vi "SCT Start Attributes Message.vi"(4 "main loop broadcast listener":T7, 6 "feature pack info":T8, 8 "error in (no error)":errorcluster, 9 "Event Registration Refnum":refnum<event-registration>, 10 "state variables in":T2, 11 "Variable Dialog Controls":T1) -> (0 "error out":errorcluster, 1 "Event Registration Refnum 2":refnum<event-registration>, 2 "state variables out":T2, 3 "Variable Dialog Controls out":T1, 5 "done?":bool)   [LabVIEW 2016]
uses:
  <resource>/dialog/variable/SCT Variable Dialog Controls.ctl
  <resource>/dialog/variable/SCT Feature Pack Info.ctl
  <resource>/dialog/variable/SCT Message User Event.ctl
  <resource>/dialog/variable/SCT Message.ctl
  <vilib>/variable/Type Descriptor.ctl
  <resource>/dialog/variable/SCT Attributes.ctl
  <resource>/dialog/variable/SCT Attributes Event.ctl
  <resource>/dialog/variable/SCT Broadcast User Event.ctl
  <resource>/dialog/variable/SCT Broadcast.ctl
  <resource>/dialog/variable/SCT State Variables.ctl
  <resource>/dialog/variable/SCT Feature State.ctl
  <resource>/dialog/variable/SCT Variable Changes.ctl
  <resource>/dialog/variable/SCT Attribute Changes.ctl
  <vilib>/variable/NI_Variable.lvlib
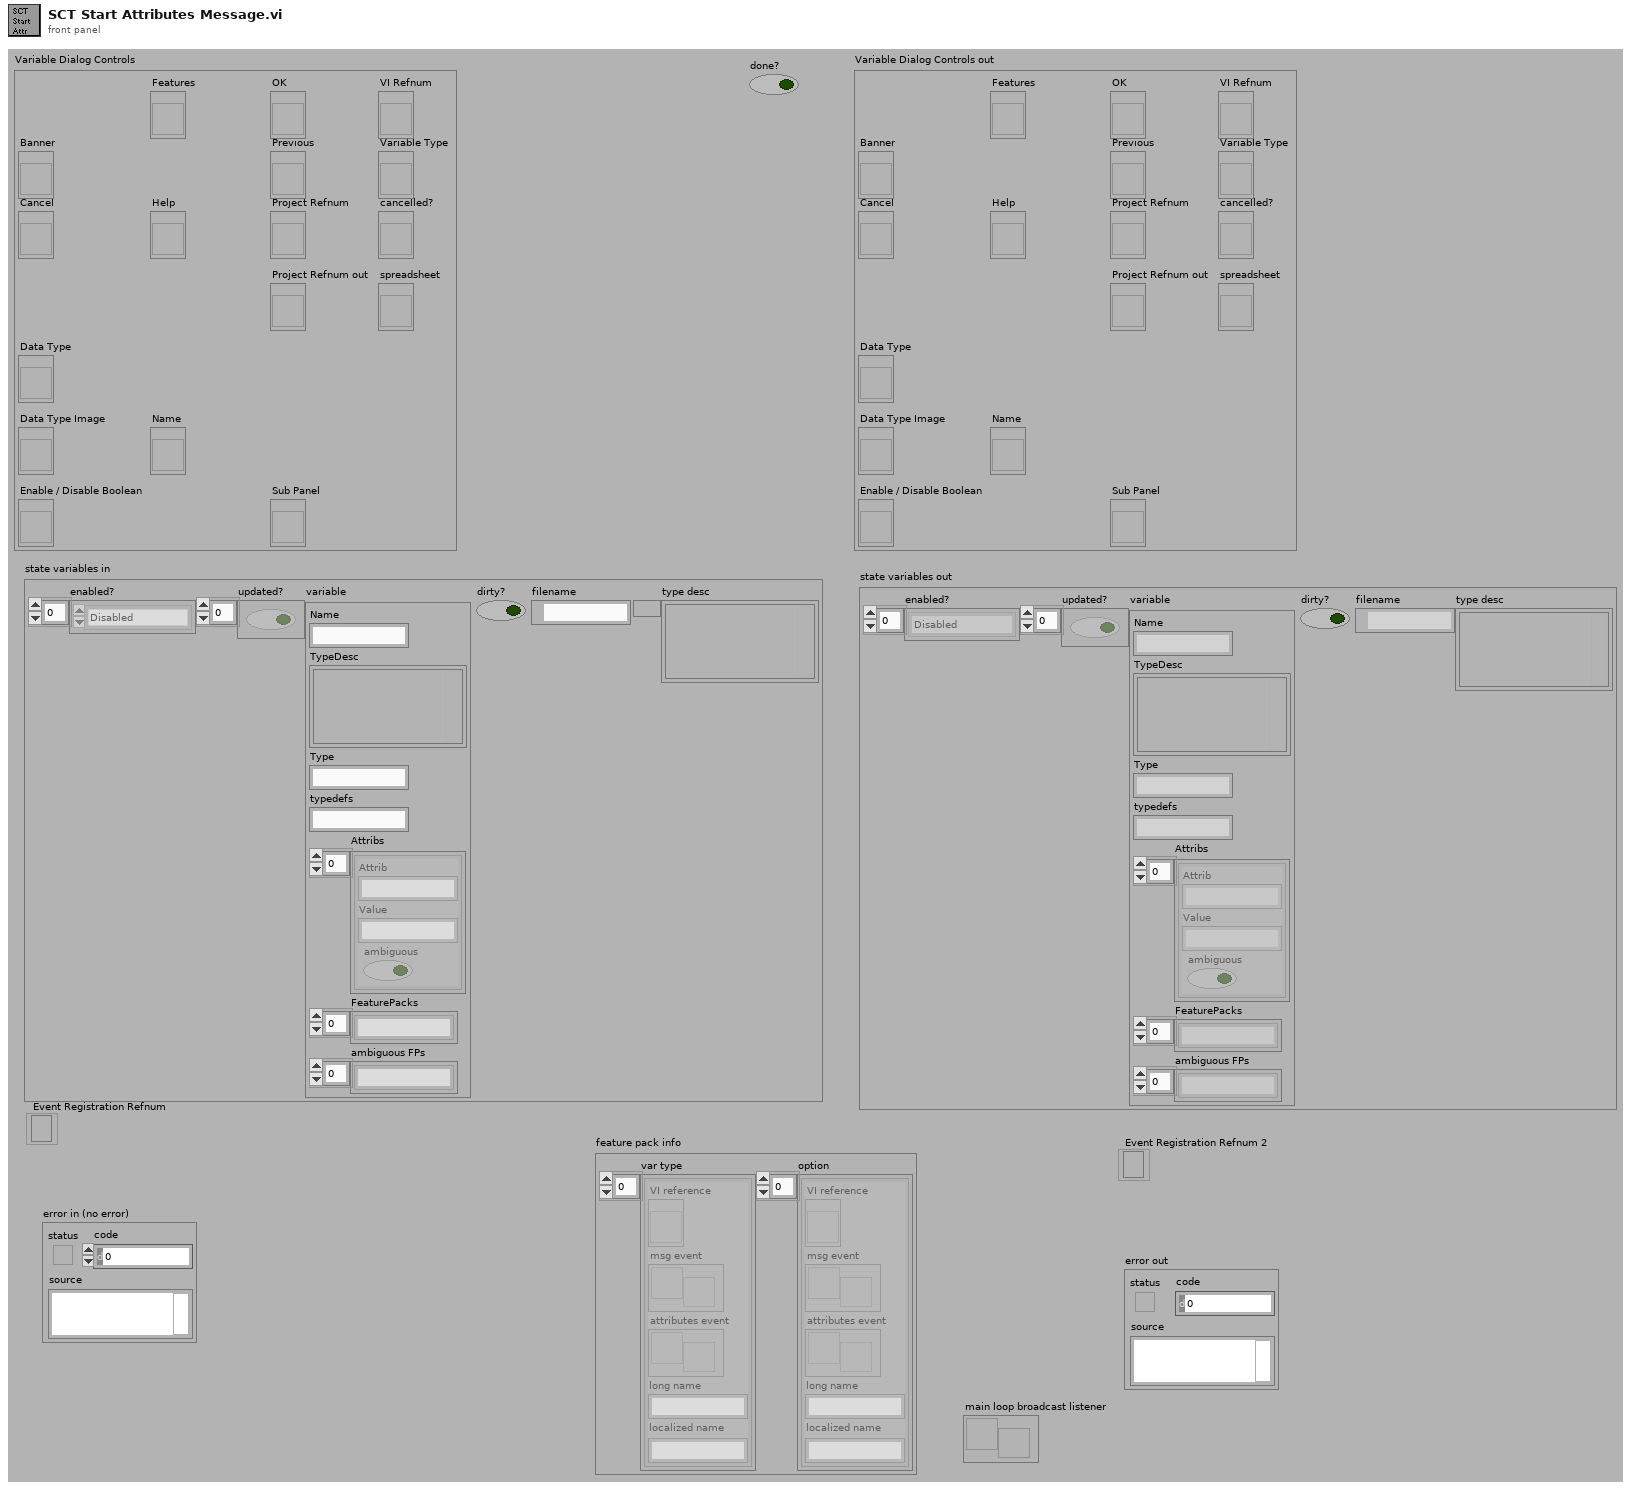
[diagram p1: front panel]
types:
  T1 = typedef "SCT Variable Dialog Controls.ctl" = cluster{"Banner":refnum<vi>, "Cancel":refnum<vi>, "Data Type":refnum<vi>, "Data Type Image":refnum<vi>, "Enable / Disable Boolean":refnum<vi>, "Features":refnum<vi>, "Help":refnum<vi>, "Name":refnum<vi>, "OK":refnum<vi>, "Previous":refnum<vi>, "Project Refnum":refnum<vi>, "Project Refnum out":refnum<vi>, "Sub Panel":refnum<vi>, "VI Refnum":refnum<vi>, "Variable Type":refnum<vi>, "cancelled?":refnum<vi>, "spreadsheet":refnum<vi>}
  T2 = typedef "SCT State Variables.ctl" = cluster{"enabled?":T3[], "updated?":bool[], "variable":T4, "dirty?":bool, "filename":path, "type desc":T5}
  T3 = typedef "SCT Feature State.ctl" = enum16{"Disabled", "Enabled", "Ambiguous", "Grayed", "MultiSelectConst"}
  T4 = typedef "SCT Variable Changes.ctl" = cluster{"Name":string, "TypeDesc":T5, "Type":string, "typedefs":string, "Attribs":T6, "FeaturePacks":string[], "ambiguous FPs":string[]}
  T5 = typedef "NI_Variable.lvlib/Type Descriptor.ctl" = cluster{"Variant":variant}
  T6 = typedef "SCT Attribute Changes.ctl" = cluster{"Attrib":string, "Value":string, "ambiguous":bool}[]
  T7 = typedef "SCT Broadcast User Event.ctl" = refnum<user-event>
  T8 = typedef "SCT Feature Pack Info.ctl" = cluster{"var type":cluster{"VI reference":refnum<vi>, "msg event":T9, "attributes event":T10, "long name":string, "localized name":string}[], "option":cluster{"VI reference":refnum<vi>, "msg event":T9, "attributes event":T10, "long name":string, "localized name":string}[]}
  T9 = typedef "SCT Message User Event.ctl" = refnum<user-event>
  T10 = typedef "SCT Attributes Event.ctl" = refnum<user-event>
  T11 = cluster{"VI reference":refnum<vi>, "msg event":T9, "attributes event":T10, "long name":string, "localized name":string}[]
  T12 = cluster{"VI reference":refnum<vi>, "msg event":T9, "attributes event":T10, "long name":string, "localized name":string}
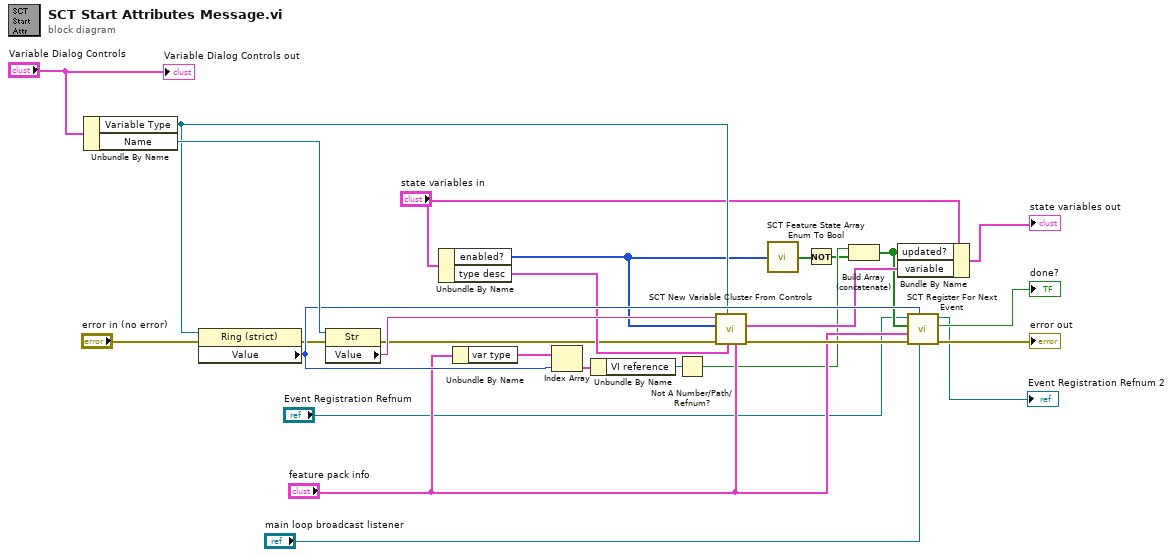
[diagram p0: block diagram]
diagram:
  n1 = Unbundle By Name("Variable Dialog Controls") -> ("Variable Type"=w24:refnum<vi>, "Name"=w26:refnum<vi>)
  n2 = property class="Ring (strict)"(reference=w24, error in="error in (no error)") -> (error out=w3:errorcluster, "Value"=w25:i32)  [unwired: 1 out]
  n3 = property class="Str"(reference=w26, error in=w3) -> (error out=w2:errorcluster, "Value"=w27:string)  [unwired: 1 out]
  n4 = Unbundle By Name("state variables in") -> ("enabled?"=w19:T3[], "type desc"=w16:T5)
  n5 = Unbundle By Name("feature pack info") -> ("var type"=w7:T11)
  n6 = Index Array(array=w7, index=w25) -> (element=w8:T12)
  n7 = Unbundle By Name(w8) -> ("VI reference"=w9:refnum<vi>)
  n8 = Not A Number/Path/Refnum?(number/path/refnum=w9) -> (NaN/Path/Refnum?=w12:bool)
  n9 = call <resource>:"SCT New Variable Cluster From Controls.vi"("feature pack info"="feature pack info", "type descriptor"=w16, "variable type ref"=w24, "error in (no error)"=w2, "enabled array"=w19, "name"=w27) -> ("error out"=w21:errorcluster, "variable"=w15:T4)  [unwired: 4 in]
  n10 = call <resource>:"SCT Feature State Array Enum To Bool.vi"("state []"=w19) -> ("enabled []"=w13:bool[])  [unwired: 4 in]
  n11 = Not(x=w13) -> (.not. x?=w11:bool[])
  n12 = Build Array (concatenate)(w12, w11) -> (w10:bool[])
  n13 = Bundle By Name(cluster="state variables in", "updated?"=w10, "variable"=w15) -> (→"state variables out":T2)
  n14 = call <resource>:"SCT Register For Next Event.vi"("main loop broadcast listener"="main loop broadcast listener", "var type index"=w25, "error in (no error)"=w21, "feature pack info"="feature pack info", "updated?"=w10, "Event Registration Refnum in"="Event Registration Refnum") -> ("error out"=→"error out":errorcluster, "done?"=→"done?":bool, "Event Registration Refnum out"=→"Event Registration Refnum 2":refnum<event-registration>)  [unwired: 3 in]
  "Variable Dialog Controls out" <- "Variable Dialog Controls"
